vi "DummyFileName.vi"(6 "Function":string, 8 "error in (no error)":errorcluster, 9 "Time String in":string) -> (0 "error out":errorcluster, 1 "Time String out":string)   [LabVIEW 2015, in "Exposure Process.lvlib"]
uses:
  Exposure Process.lvlib
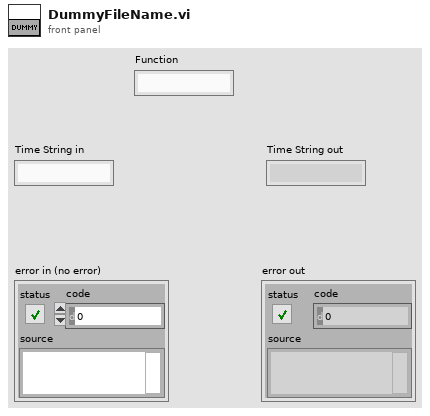
[diagram p1: front panel]
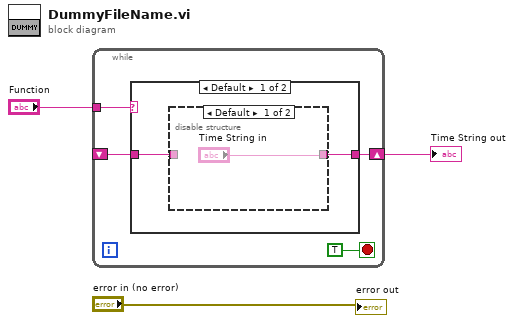
[diagram p0: block diagram]
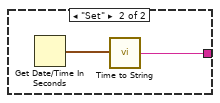
[diagram p3: hidden frame]
diagram:
  n1 = while {
    tunnel: "Function" -> [w7]
    shift-right: [w6] -> w1
    shift-left: _ -> [w5]
    stop <- TRUE stop-if-true
    n2 = case shown="Default" w7 {
      tunnel: [w8 w12] -> w6
      tunnel: w5 -> [w9 _]
      frame Default {
        n3 = disable-structure shown="Default" {
          disable-tunnel: w9 -> [_ w11]
          disable-tunnel: ["Time String in" w11] -> w8
          frame condition #0 {
          }
          frame condition #1 (active) {
          }
        }
      }
      frame "Set" {
        n4 = Get Date/Time In Seconds() -> (seconds since 1Jan1904=w13:timestamp)
        n5 = call "Time to String.vi"("Time Stamp"=w13) -> ("date/time string"=w12:string)
      }
    }
  }
  "Time String out" <- w1
  "error out" <- "error in (no error)"
